vi "stat_f_s1.vi"(6 "kD":sgl=1.3, 7 "Y":i16[](array[numeric])) -> (1 "stops":i32[](array[numeric]), 2 "starts":i32[](array[numeric]), 3 "mean":dbl format="%0.2f")   [LabVIEW 2010]
panel:
  out "Array":i32[](array[numeric])
  out "Waveform Graph":cluster{"Numeric":i32, i32, i16[]}(graph)
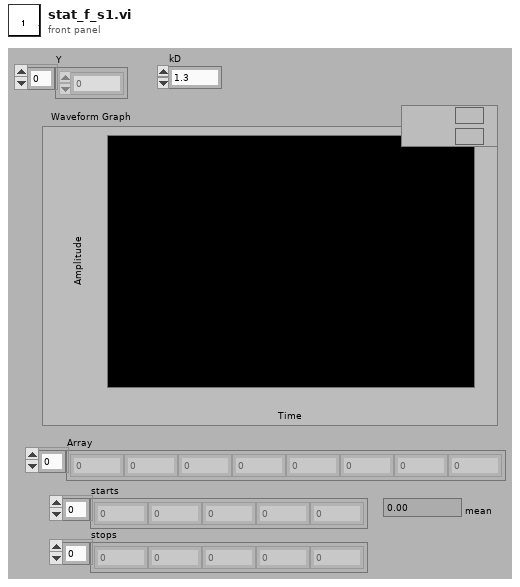
[diagram p1: front panel]
types:
  T1 = cluster{"Name":string, "Color":u32, "Style":u8, "Point Style":u8, "Name Visible":bool, "Allow Drag":bool, "Lock Style":u32, "Plot":u32, "Index":i32, "Position":cluster{"X":dbl, "Y":dbl}}[]
  T2 = cluster{"Name":string, "Color":u32, "Style":u8, "Point Style":u8, "Name Visible":bool, "Allow Drag":bool, "Lock Style":u32, "Plot":u32, "Index":i32, "Position":cluster{"X":dbl, "Y":dbl}}
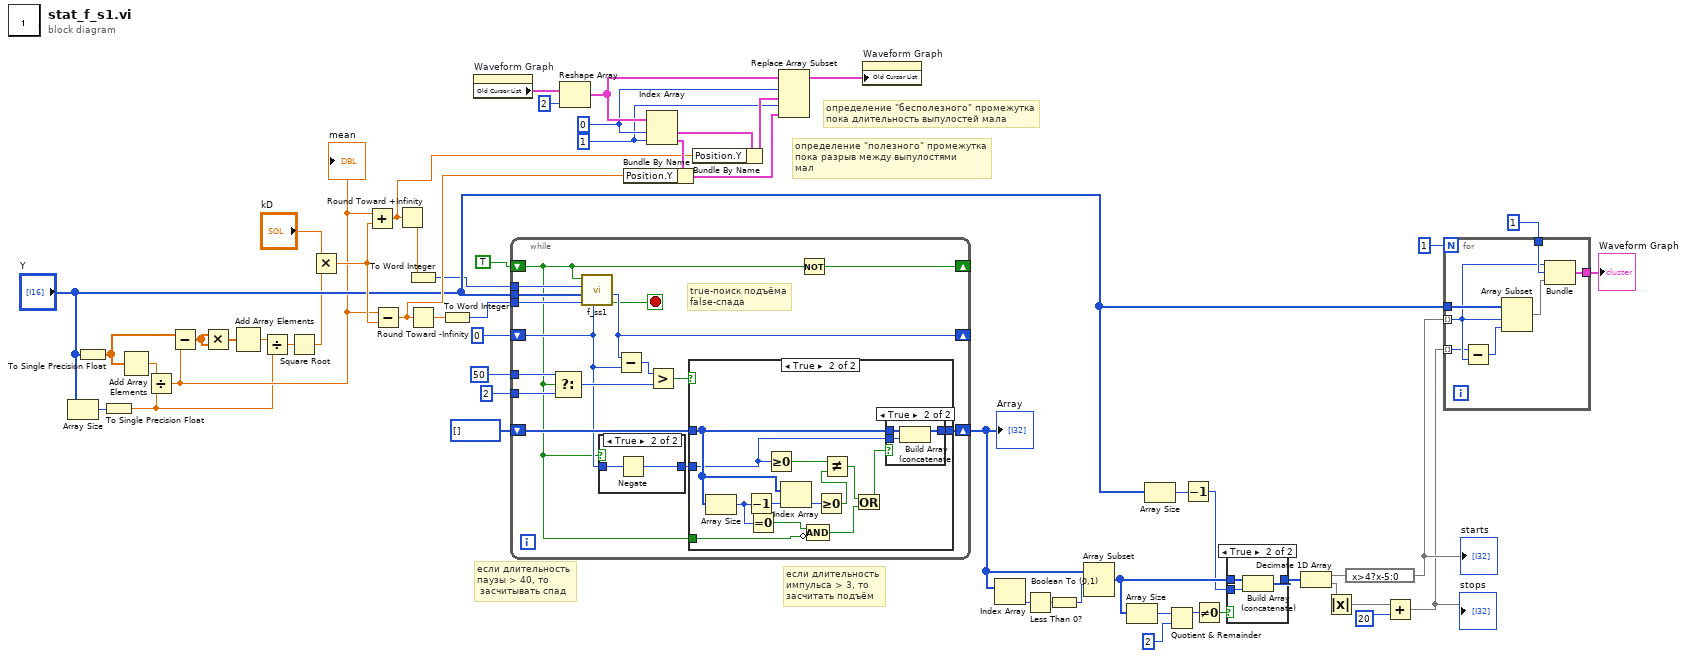
[diagram p0: block diagram]
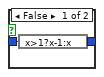
[diagram p3: hidden frame]
diagram:
  w46 = 1 ("index")
  w47 = 0 ("index")
  # "если длительность\nимпульса > 3, то\nзасчитать подъём"
  # "если длительность\nпаузы > 40, то\n засчитывать спад"
  # "определение \"полезного\" промежутка\nпока разрыв между выпулостями\nмал"
  # "определение \"бесполезного\" промежутка\nпока длительность выпулостей мала"
  n1 = Array Size(array="Y") -> (size(s)=w6:i32)
  n2 = To Single Precision Float(number="Y") -> (single precision float=w7:sgl[])
  n3 = To Single Precision Float(number=w6) -> (single precision float=w5:sgl)
  n4 = Add Array Elements(numeric array=w7) -> (sum=w13:sgl)
  n5 = Divide(x=w13, y=w5) -> (x/y=w11:sgl)
  "mean" <- w11
  n6 = Subtract(x=w7, y=w11) -> (x-y=w10:sgl[])
  n7 = Multiply(x=w10, y=w10) -> (x*y=w9:sgl[])
  n8 = Add Array Elements(numeric array=w9) -> (sum=w8:sgl)
  n9 = Divide(x=w8, y=w5) -> (x/y=w4:sgl)
  n10 = Square Root(x=w4) -> (sqrt(x)=w3:sgl)
  n11 = Multiply(x="kD", y=w3) -> (x*y=w40:sgl)
  n12 = Add(x=w11, y=w40) -> (x+y=w17:sgl)
  n13 = Subtract(x=w11, y=w40) -> (x-y=w16:sgl)
  n14 = Round Toward +Infinity(x=w17) -> (ceil(x): smallest int >= x=w14:sgl)
  n15 = To Word Integer(number=w14) -> (16bit integer=w1:i16)
  n16 = Round Toward -Infinity(1:w16) -> (0:w15:sgl)
  n17 = To Word Integer(number=w15) -> (16bit integer=w2:i16)
  n18 = property on="Waveform Graph" class="WFGraph (strict)"() -> ("Old Cursor List"=w55:T1)  [unwired: 2 in, 2 out]
  n19 = while {
    tunnel: w2 -> [w68]
    tunnel: w1 -> [w69]
    tunnel: "Y" -> [w70]
    shift-right: [w66] -> _
    shift-left: 0 -> [w58]
    shift-right: [w67] -> _
    shift-left: TRUE ("Boolean") -> [w56]
    tunnel: 50 ("t") -> [w63]
    tunnel: 2 -> [w62]
    shift-right: [w60] -> w34
    shift-left: i32[] [] -> [w59]
    stop <- w65 stop-if-true
    # "true-поиск подъёма\nfalse-спада"
    n20 = Select(t=w63, s=w56, f=w62) -> (s? t:f=w61:i32)
    n21 = call "f_ss1.vi"("index in"=w58, "lower lim"=w68, "Y"=w70, "upper lim"=w69, "Boolean"=w56) -> ("eof"=w65:bool, "index out"=w66:i32)  [unwired: 1 in, 1 out]
    n22 = case shown="True" w56 {
      tunnel: [w73 w74] -> w57
      tunnel: w58 -> [w72 w75]
      frame False {
        n23 = expression code="x>1?x-1:x"(w72) -> (w73:i32)
      }
      frame True {
        n24 = Negate(x=w75) -> (-x=w74:i32)
      }
    }
    n25 = Subtract(x=w66, y=w58) -> (x-y=w71:i32)
    n26 = Greater?(x=w71, y=w61) -> (0:w64:bool)
    n27 = case shown="True" w64 {
      tunnel: w57 -> [_ w85]
      tunnel: [w76 w89] -> w60
      tunnel: w59 -> [w76 w87]
      tunnel: w56 -> [_ w78]
      frame False {
      }
      frame True {
        n28 = Array Size(array=w87) -> (size(s)=w82:i32)
        n29 = Decrement(x=w82) -> (x-1=w88:i32)
        n30 = Equal To 0?(x=w82) -> (x = 0?=w79:bool)
        n31 = Greater Or Equal To 0?(x=w85) -> (x >= 0?=w83:bool)
        n32 = Index Array(array=w87, index=w88) -> (element=w86:i32)
        n33 = Compound Arithmetic op=AND(w79, invert w78) -> (w77:bool)
        n34 = Greater Or Equal To 0?(x=w86) -> (x >= 0?=w84:bool)
        n35 = Not Equal?(x=w83, y=w84) -> (x != y?=w81:bool)
        n36 = Or(x=w81, y=w77) -> (x .or. y?=w80:bool)
        n37 = case shown="True" w80 {
          tunnel: w85 -> [_ w93]
          tunnel: [w90 w92] -> w89
          tunnel: w87 -> [w90 w91]
          frame False {
          }
          frame True {
            n38 = Build Array (concatenate)(w91, w93) -> (w92:i32[])
          }
        }
      }
    }
    n39 = Not(x=w56) -> (.not. x?=w67:bool)
  }
  "Array" <- w34
  n40 = Reshape Array(w55, 2 ("dimension size")) -> (w51:T1)
  n41 = Index Array(array=w51, index #1=w47, index #2=w46) -> (element #1=w53:T2, element #2=w52:T2)
  n42 = Bundle By Name(cluster=w52, "Position.Y"=w16) -> (w49:T2)
  n43 = Bundle By Name(cluster=w53, "Position.Y"=w17) -> (w50:T2)
  n44 = Replace Array Subset(array=w51, new element #1=w50, index #1=w47, new element #2=w49, index #2=w46) -> (w48:T1)
  n45 = property on="Waveform Graph" class="WFGraph (strict)"("Old Cursor List"=w48) -> ()  [unwired: 2 in, 2 out]
  n46 = Index Array(array=w34) -> (element=w38:i32)  [unwired: 1 in]
  n47 = Less Than 0?(x=w38) -> (x < 0?=w37:bool)
  n48 = Boolean To (0,1)(Boolean=w37) -> (0, 1=w36:i16)
  n49 = Array Subset(array=w34, index=w36) -> (w30:i32[])  [unwired: 1 in]
  n50 = Array Size(array=w30) -> (size(s)=w29:i32)
  n51 = Array Size(array="Y") -> (size(s)=w26:i32)
  n52 = Quotient & Remainder(x=w29, y=2) -> (x-y*floor(x/y)=w32:i32)  [unwired: 1 out]
  n53 = Decrement(x=w26) -> (x-1=w28:i32)
  n54 = Not Equal To 0?(x=w32) -> (x != 0?=w31:bool)
  n55 = case shown="True" w31 {
    tunnel: w30 -> [w94 w97]
    tunnel: w28 -> [_ w96]
    tunnel: [w94 w95] -> w27
    frame False {
    }
    frame True {
      n56 = Build Array (concatenate)(w97, w96) -> (w95:i32[])
    }
  }
  n57 = Decimate 1D Array(w27) -> (w25:i32[], w35:i32[])
  n58 = Absolute Value(x=w35) -> (abs(x)=w20:i32[])
  n59 = expression code="x>4?x-5:0"(w25) -> (w21:i32[])
  "starts" <- w21
  n60 = Add(x=w20, y=20) -> (x+y=w18:i32[])
  "stops" <- w18
  n61 = for {
    N: 1 -> [_]
    tunnel: w21 -> [w100] mode=indexing
    tunnel: "Y" -> [w104]
    tunnel: w18 -> [w99] mode=indexing
    tunnel: 1 -> [w102]
    tunnel: [w101] -> w23
    n62 = Subtract(x=w99, y=w100) -> (x-y=w98:i32)
    n63 = Array Subset(array=w104, index=w100, length=w98) -> (w103:i16[])
    n64 = Bundle("Numeric"=w100, w102, w103) -> (w101:cluster{"Numeric":i32, i32, i16[]})  [unwired: 1 in]
  }
  "Waveform Graph" <- w23
